vi "Generate Test Case.vi"(8 "error in (no error)":errorcluster, 11 "Process Generator In":refnum<class "Process Generator.lvclass">) -> (0 "error out":errorcluster, 3 "Process Generator Out":refnum<class "Process Generator.lvclass">)   [LabVIEW 2020, in "Process Generation.lvlib" / "Process Generator.lvclass"]
uses:
  Process Generator.lvclass
  Process Generator.lvclass/Process Generator.ctl
  Framework Test Suite/Process Test/Process Test.lvclass
  <vilib>/Utility/traverseref.llb/TRef TravTarget.ctl
  <vilib>/Utility/traverseref.llb/VI Scripting - Traverse.lvlib
  <vilib>/Astemes/LUnit/Test Case.lvclass
  C:/Git/astemes-triarc-framework/source/Framework Test Suite/Base Class Test/Base Test.lvclass
  C:/Program Files (x86)/National Instruments/LabVIEW 2020/vi.lib/Astemes/LUnit/Test Case.lvclass
  C:/Git/astemes-triarc-framework/source/Framework Test Suite/Process Test/Process Test.lvclass
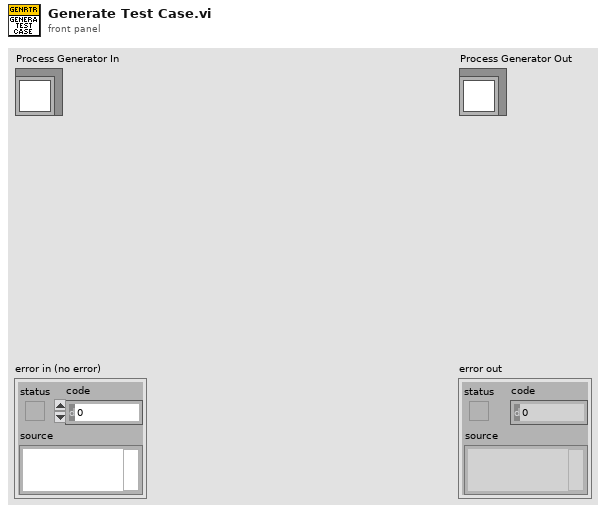
[diagram p1: front panel]
types:
  T1 = typedef "TRef TravTarget.ctl" = enum16{"FP", "BD", "Other"}
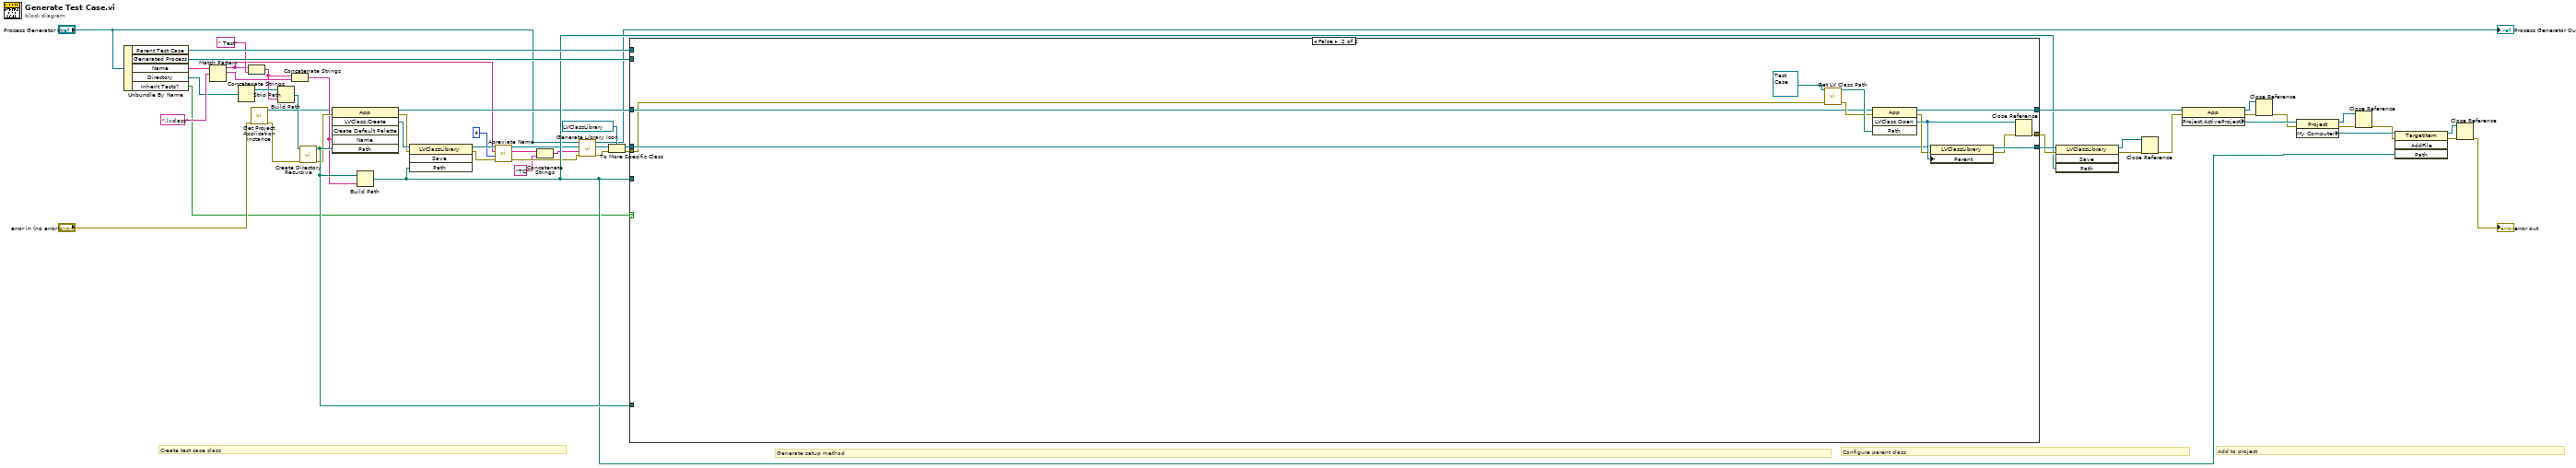
[diagram p0: block diagram]
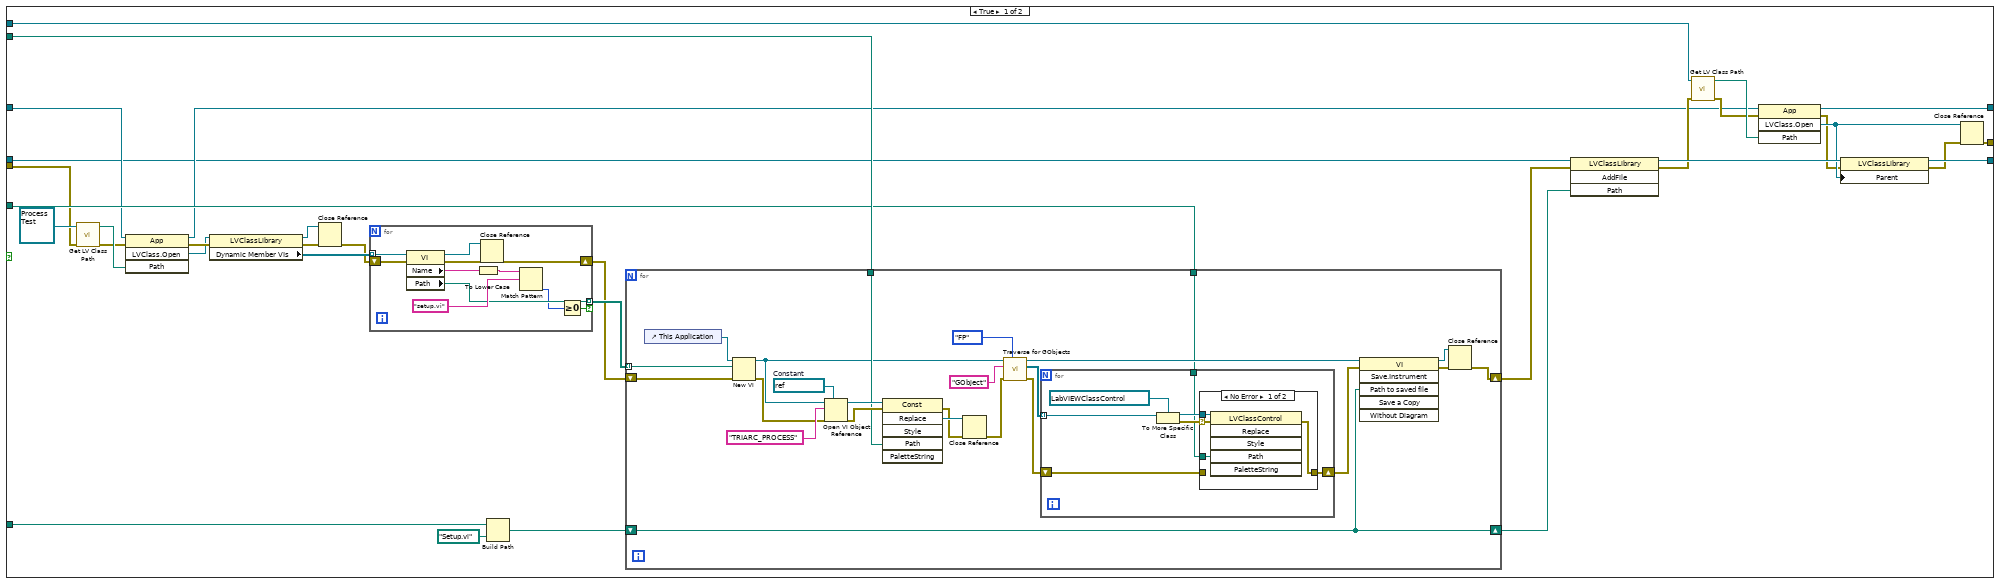
[diagram p2: hidden frame]
diagram:
  # "Add to project"
  # "Configure parent class"
  # "Create test case class"
  # "Generate setup method"
  n1 = Unbundle By Name("Process Generator In") -> ("Parent Test Case"=w53:refnum<class "Test Case.lvclass">, "Generated Process"=w38:path, "Name"=w30:string, "Directory"=w27:path, "Inherit Tests?"=w1:bool)
  n2 = Match Pattern(string=w30, regular expression=".lvclass" ("string")) -> (before substring=w8:string, match substring=w25:string)  [unwired: 1 in, 2 out]
  n3 = Strip Path(path=w27) -> (stripped path=w24:path)  [unwired: 1 out]
  n4 = Concatenate Strings(w8, " Test" ("string")) -> (w23:string)
  n5 = call "Get Project Application Instance.vi"("error in (no error)"="error in (no error)") -> ("error out"=w19:errorcluster, "Application out"=w21:refnum<vi>)  [unwired: 9 in]
  n6 = Build Path(base path=w24, name or relative path=w23) -> (appended path=w22:path)
  n7 = Concatenate Strings(w23, w25) -> (w26:string)
  n8 = call <vilib>:"Create Directory Recursive.vi"("error in (no error)"=w19, "directory"=w22) -> ("error out"=w36:errorcluster, "directory copy"=w37:path)  [unwired: 3 in, 1 out]
  n9 = invoke class="App" method="LVClass.Create"(reference=w21, error in=w36, "Name"=w26, "Path"=w37) -> (reference out=w17:refnum<vi>, error out=w18:errorcluster, "LVClass.Create"=w32:refnum<vi>)  [unwired: 2 in, 3 out]
  n10 = Build Path(base path=w37, name or relative path=w26) -> (appended path=w31:path)
  n11 = invoke class="LVClassLibrary" method="Save"(reference=w32, error in=w18, "Path"=w31) -> (reference out=w13:refnum<vi>, error out=w11:errorcluster)  [unwired: 1 in, 2 out]
  n12 = call "Abreviate Name.vi"("error in (no error)"=w11, "Max Length"=4, "Long Name"=w8) -> ("error out"=w10:errorcluster, "Abreviated Name"=w6:string)  [unwired: 7 in]
  n13 = Concatenate Strings(w6, "TC" ("string")) -> (w5:string)
  n14 = call "Generate Library Icon.vi"("error in (no error)"=w10, "Overlay Text"=w5, "Library"=w13, "Process Generator In"="Process Generator In") -> ("error out"=w14:errorcluster, "Library Out"=w16:refnum<vi>, "Process Generator Out"=→"Process Generator Out":refnum<class "Process Generator.lvclass">)  [unwired: 5 in]
  n15 = To More Specific Class(target class=refnum<vi> refnum ("reference out"), reference=w16, error in=w14) -> (specific class reference=w12:refnum<vi>, error out=w9:errorcluster)
  n16 = case shown="False" w1 {
    tunnel: w53 -> [w86 _]
    tunnel: [w84 w144] -> w52
    tunnel: w38 -> [w78 _]
    tunnel: w37 -> [w76 _]
    tunnel: [w71 w142] -> w34
    tunnel: [w69 w140] -> w33
    tunnel: w31 -> [w68 _]
    tunnel: w17 -> [w61 w137]
    tunnel: w12 -> [w55 w136]
    tunnel: w9 -> [w54 w135]
    frame True {
      n17 = call <vilib>:"Get LV Class Path.vi"("error in (no error)"=w54, "object"=refnum<class "Process Test.lvclass"> refnum ("Process Test.lvclass")) -> ("error out"=w62:errorcluster, "class path"=w63:path)  [unwired: 8 in]
      n18 = invoke class="App" method="LVClass.Open"(reference=w61, error in=w62, "Path"=w63) -> (reference out=w60:refnum<vi>, error out=w59:errorcluster, "LVClass.Open"=w58:refnum<vi>)  [unwired: 1 in, 1 out]
      n19 = property class="LVClassLibrary"(reference=w58, error in=w59) -> (reference out=w56:refnum<vi>, error out=w79:errorcluster, "Dynamic Member VIs"=w82:refnum<vi>[])
      n20 = Close Reference(reference=w56, error in (no error)=w79) -> (error out=w57:errorcluster)
      n21 = for {
        tunnel: w82 -> [w133] mode=indexing
        shift-right: [w126] -> w80
        shift-left: w57 -> [w129]
        tunnel: [w127] -> w81 mode=indexing if=w124
        n22 = property class="VI"(reference=w133, error in=w129) -> (reference out=w125:refnum<vi>, error out=w128:errorcluster, "Name"=w132:string, "Path"=w127:path)
        n23 = To Lower Case(string=w132) -> (all lower case string=w131:string)
        n24 = Close Reference(reference=w125, error in (no error)=w128) -> (error out=w126:errorcluster)
        n25 = Match Pattern(string=w131, regular expression="setup.vi" ("y")) -> (offset past match=w123:i32)  [unwired: 1 in, 3 out]
        n26 = Greater Or Equal To 0?(x=w123) -> (x >= 0?=w124:bool)
      }
      n27 = Build Path(base path=w76, name or relative path=path "Setup.vi") -> (appended path=w74:path)
      n28 = for {
        tunnel: w81 -> [w110] mode=indexing
        shift-right: [w99] -> w77
        shift-left: w80 -> [w109]
        tunnel: w78 -> [w103]
        tunnel: w68 -> [w90]
        shift-right: [w97] -> w73
        shift-left: w74 -> [w97]
        w107 = refnum<vi> refnum  # Constant
        n29 = control-ref of="This Application"() -> (w87:refnum<vi>)
        n30 = New VI(8:w109, 10:w110, 11:w87) -> (0:w106:errorcluster, 3:w96:refnum<vi>)  [unwired: 4 in]
        n31 = Open VI Object Reference(7:w107, 8:w106, 10:"TRIARC_PROCESS" ("name/order"), 11:w96) -> (0:w104:errorcluster, 3:w105:refnum<vi>)
        n32 = invoke on="Invoke Node" class="Const" method="Replace"(reference=w105, error in=w104, "Path"=w103) -> (error out=w101:errorcluster, "Replace"=w102:refnum<vi>)  [unwired: 3 in, 4 out]
        n33 = Close Reference(reference=w102, error in (no error)=w101) -> (error out=w92:errorcluster)
        n34 = call <vilib>:"Traverse for GObjects.vi"("Traverse Target"=TRef_TravTarget."FP", "error in (no error)"=w92, "Class Name"="GObject", "VI Refnum"=w96) -> ("error out"=w88:errorcluster, "References"=w91:refnum<vi>[], "dup VI Refnum"=w95:refnum<vi>)  [unwired: 4 in, 1 out]
        n35 = for {
          tunnel: w91 -> [w117] mode=indexing
          tunnel: w90 -> [w113]
          shift-right: [w112] -> w89
          shift-left: w88 -> [w111]
          n36 = To More Specific Class(target class=refnum<vi> refnum ("reference out"), reference=w117) -> (specific class reference=w114:refnum<vi>, error out=w115:errorcluster)  [unwired: 1 in]
          n37 = case shown="No Error" w115 {
            selector: w115 -> [w121 _]
            tunnel: w114 -> [w120 _]
            tunnel: w113 -> [w119 _]
            tunnel: [w118 w122] -> w112
            tunnel: w111 -> [_ w122]
            frame No Error {
              n38 = invoke on="Invoke Node" class="LVClassControl" method="Replace"(reference=w120, error in=w121, "Path"=w119) -> (error out=w118:errorcluster)  [unwired: 3 in, 5 out]
            }
            frame Error {
            }
          }
        }
        n39 = invoke on="Invoke Node" class="VI" method="Save.Instrument"(reference=w95, error in=w89, "Path to saved file"=w97) -> (reference out=w98:refnum<vi>, error out=w100:errorcluster)  [unwired: 3 in, 4 out]
        n40 = Close Reference(reference=w98, error in (no error)=w100) -> (error out=w99:errorcluster)
      }
      n41 = invoke class="LVClassLibrary" method="AddFile"(reference=w55, error in=w77, "Path"=w73) -> (reference out=w72:refnum<vi>, error out=w66:errorcluster)  [unwired: 1 in, 2 out]
      n42 = call <vilib>:"Get LV Class Path.vi"("error in (no error)"=w66, "object"=w86) -> ("error out"=w83:errorcluster, "class path"=w85:path)  [unwired: 8 in]
      n43 = invoke class="App" method="LVClass.Open"(reference=w60, error in=w83, "Path"=w85) -> (reference out=w84:refnum<vi>, error out=w65:errorcluster, "LVClass.Open"=w67:refnum<vi>)  [unwired: 1 in, 1 out]
      n44 = property class="LVClassLibrary"(reference=w72, error in=w65, "Parent"=w67) -> (reference out=w71:refnum<vi>, error out=w70:errorcluster)
      n45 = Close Reference(reference=w67, error in (no error)=w70) -> (error out=w69:errorcluster)
    }
    frame False {
      n46 = call <vilib>:"Get LV Class Path.vi"("error in (no error)"=w135, "object"=refnum<class "Test Case.lvclass"> refnum ("Test Case.lvclass")) -> ("error out"=w143:errorcluster, "class path"=w145:path)  [unwired: 8 in]
      n47 = invoke class="App" method="LVClass.Open"(reference=w137, error in=w143, "Path"=w145) -> (reference out=w144:refnum<vi>, error out=w138:errorcluster, "LVClass.Open"=w139:refnum<vi>)  [unwired: 1 in, 1 out]
      n48 = property class="LVClassLibrary"(reference=w136, error in=w138, "Parent"=w139) -> (reference out=w142:refnum<vi>, error out=w141:errorcluster)
      n49 = Close Reference(reference=w139, error in (no error)=w141) -> (error out=w140:errorcluster)
    }
  }
  n50 = invoke class="LVClassLibrary" method="Save"(reference=w34, error in=w33, "Path"=w31) -> (reference out=w35:refnum<vi>, error out=w48:errorcluster)  [unwired: 1 in, 2 out]
  n51 = Close Reference(reference=w35, error in (no error)=w48) -> (error out=w47:errorcluster)
  n52 = property class="App"(reference=w52, error in=w47) -> (reference out=w43:refnum<vi>, error out=w50:errorcluster, "Project.ActiveProject"=w51:refnum<vi>)
  n53 = Close Reference(reference=w43, error in (no error)=w50) -> (error out=w44:errorcluster)
  n54 = property class="Project"(reference=w51, error in=w44) -> (reference out=w41:refnum<vi>, error out=w46:errorcluster, "My Computer"=w49:refnum<vi>)
  n55 = Close Reference(reference=w41, error in (no error)=w46) -> (error out=w42:errorcluster)
  n56 = invoke class="TargetItem" method="AddFile"(reference=w49, error in=w42, "Path"=w31) -> (reference out=w39:refnum<vi>, error out=w45:errorcluster)  [unwired: 1 in, 2 out]
  n57 = Close Reference(reference=w39, error in (no error)=w45) -> (error out=→"error out":errorcluster)
